vi "Test_data_read.vi"() -> ()   [LabVIEW 2018]
panel:
  in  "file (use dialog)":path=path "C:/Users/Dmitriy/Documents/MHC_Tracker/TrackTemp-2018-04-05-17-50-01.trtmp"
  out "rest of the binary string":string
  out "data":string
  out "value":T1(array[cluster])
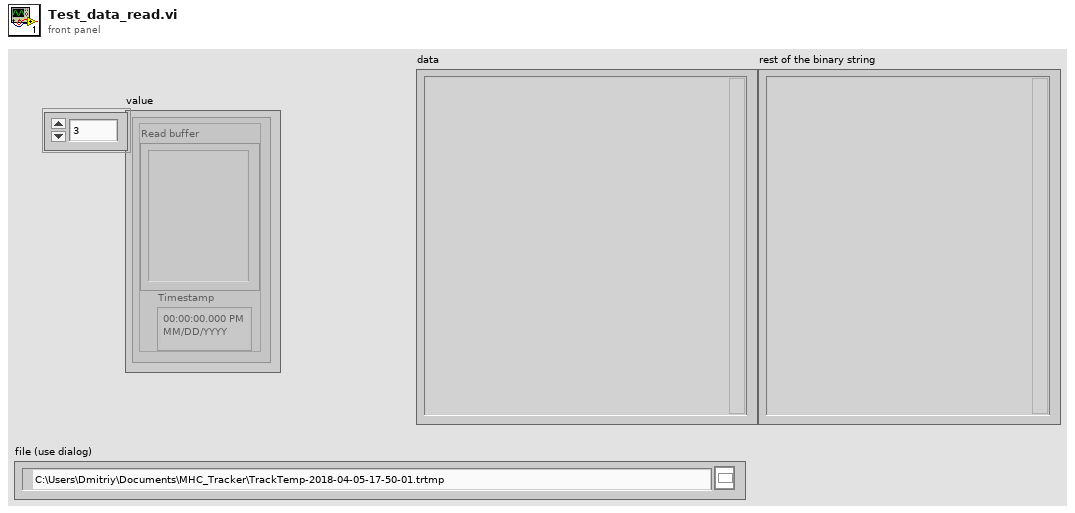
[diagram p1: front panel]
types:
  T1 = cluster{"Read buffer":string, "Timestamp":timestamp}[]
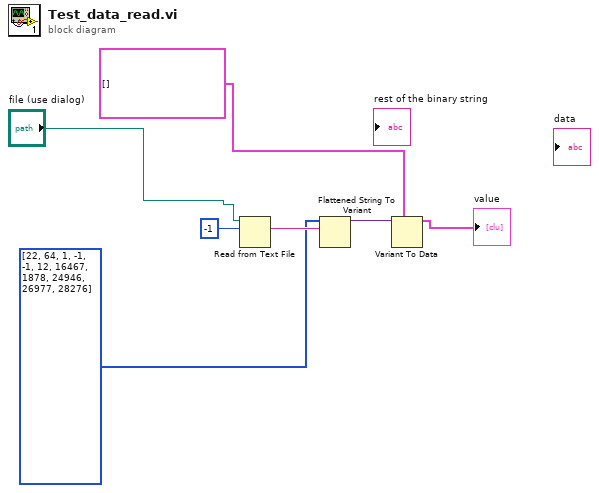
[diagram p0: block diagram]
diagram:
  n1 = Read from Text File(file (use dialog)="file (use dialog)", count=-1) -> (text=w6:string)  [unwired: 2 in, 3 out]
  n2 = Flattened String To Variant(6:w6, 7:i16[] [22, 64, 1, -1, -1, 12, 16467, 1878, 24946, 26977, 28276] ("type string")) -> (3:w4:variant)  [unwired: 1 in, 1 out]
  n3 = Variant To Data(type=T1 [], Variant=w4) -> (data=→"value":T1)  [unwired: 1 in, 1 out]
